vi "addItem.vi"(0 "reference in":refnum<class "Items Controller.lvclass">, 5 "dataIN":string[](array[string]), 7 "storageIN":string[][](array[string]), 11 "error in (no error)":errorcluster) -> (4 "reference out":refnum<class "Items Controller.lvclass">, 6 "found?":bool, 10 "storageOUT":string[][](array[string]), 15 "error out":errorcluster)   [LabVIEW 2014, in "Items Controller.lvclass"]
uses:
  Items Controller.lvclass
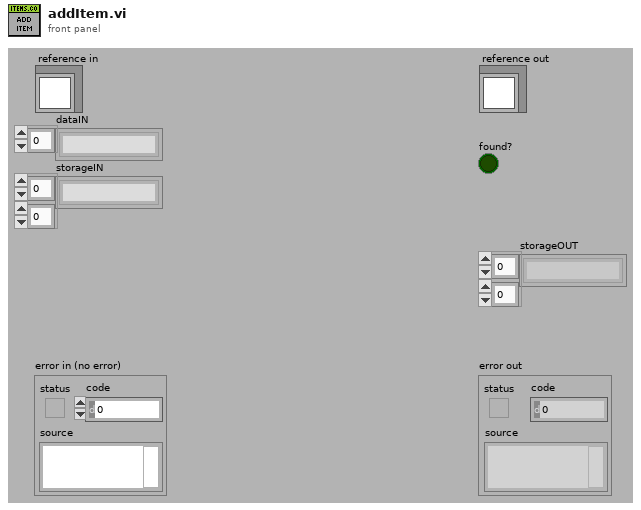
[diagram p1: front panel]
types:
  T1 = typedef "Items Controller.lvclass/ObjectAttributesRef.ctl" = refnum<data-value>
  T2 = typedef "Items Controller.lvclass/ObjectAttributes.ctl" = cluster{"MyAttribute":dbl, "data":string[][][], "file_controller_ref":refnum<class "File Controller.lvclass">, "checkIN_ref":refnum<class "checkIN.lvclass">, "checkOUT_ref":refnum<class "checkOUT.lvclass">, "item_ref":refnum<class "item.lvclass">}
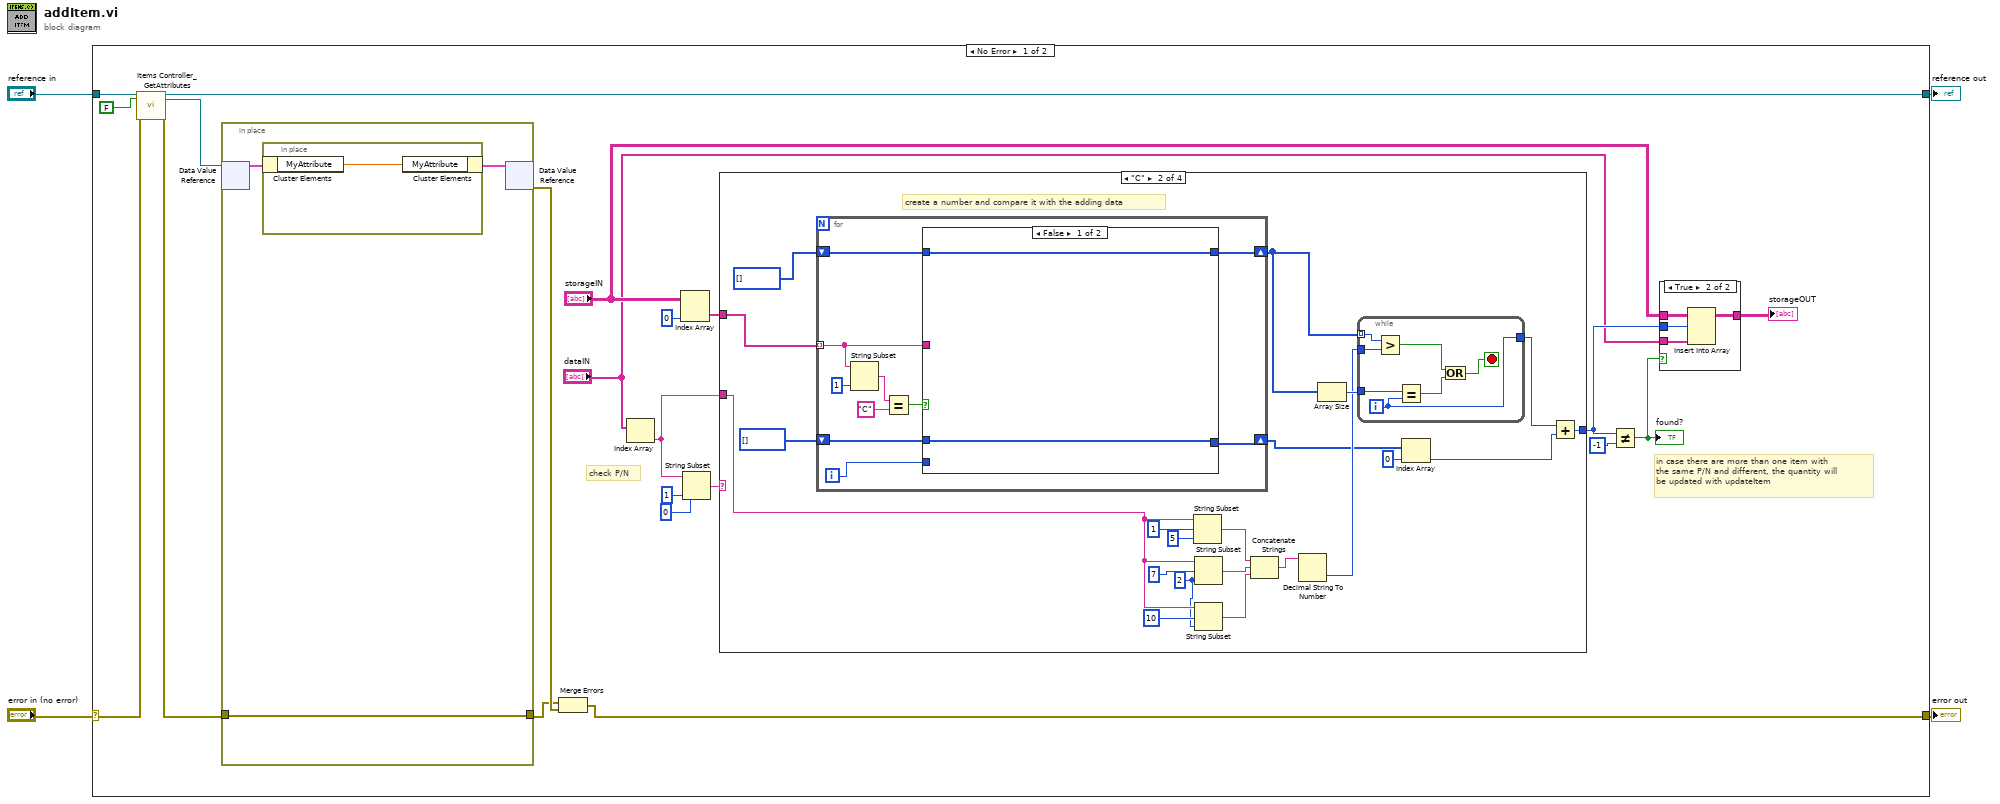
[diagram p0: block diagram]
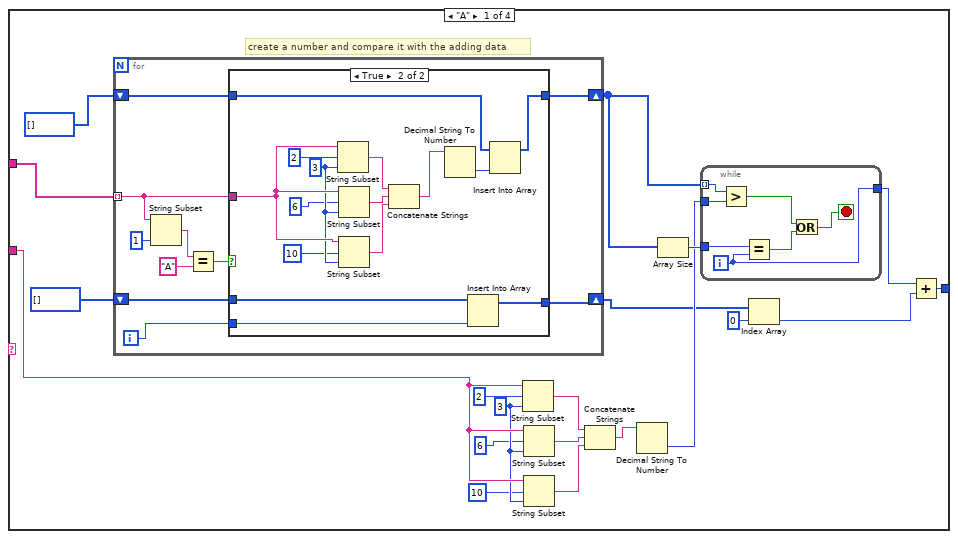
[diagram p3: hidden frame]
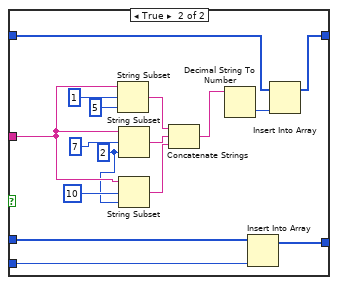
[diagram p5: hidden frame]
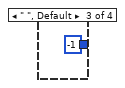
[diagram p6: hidden frame]
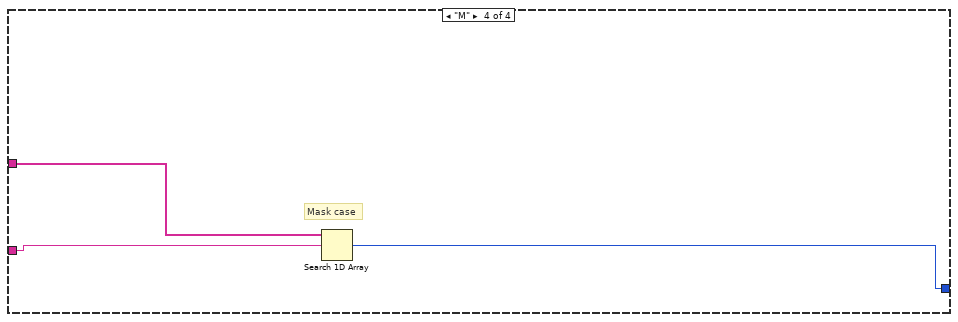
[diagram p7: hidden frame]
diagram:
  n1 = case shown="No Error" "error in (no error)" {
    selector: "error in (no error)" -> [w21 w150]
    tunnel: [w17 w150] -> w3
    tunnel: [w19 w149] -> w1
    tunnel: "reference in" -> [w23 w149]
    frame No Error {
      # "in case there are more than one item with\nthe same P/N and different, the quantity will\nbe updated with updateItem"
      # "check P/N"
      n2 = call "Items Controller_GetAttributes.vi"("reference in"=w23, "return data? (T)"=FALSE, "error in (no error)"=w21) -> ("reference out"=w19:refnum<class "Items Controller.lvclass">, "attributes ref"=w18:T1, "error out"=w20:errorcluster)  [unwired: 13 in, 1 out]
      n3 = in-place {
        in-place-border: w20 -> [w145]
        in-place-border: [w145] -> w24
        n4 = in-place-dvr #1(w18) -> (w146:T2)  [unwired: 1 out]
        n5 = in-place {
          n6 = in-place-cluster #2(w146) -> ("MyAttribute"=w148:dbl)
          n7 = in-place-cluster #2("MyAttribute"=w148) -> (w147:T2)
        }
        n8 = in-place-dvr #1(w147) -> (w25:errorcluster)  [unwired: 1 out]
      }
      n9 = Merge Errors(w24, w25) -> (w17:errorcluster)
      n10 = Index Array(array="dataIN") -> (element=w13:string)  [unwired: 1 in]
      n11 = Index Array(array="storageIN", index (col)=0 ("disabled index (col)")) -> (element=w12:string[])  [unwired: 1 in]
      n12 = String Subset(string=w13, offset (0)=0, length (rest)=1 ("length (rest)")) -> (substring=w14:string)
      n13 = case shown="\"C\"" w14 {
        tunnel: w13 -> [w50 w105 _ w143]
        tunnel: w12 -> [w49 w104 _ w144]
        tunnel: [w31 w86 -1 w142] -> w7
        frame "A" {
          w47 = 3 ("length (rest)")
          # "create a number and compare it with the adding data"
          n14 = for {
            tunnel: w49 -> [w64] mode=indexing
            shift-right: [w61] -> w38
            shift-left: i32[] [] -> [w62]
            shift-right: [w59] -> w35
            shift-left: i32[] [] -> [w60]
            i -> [w58]
            n15 = String Subset(string=w64, length (rest)=1 ("length (rest)")) -> (substring=w66:string)  [unwired: 1 in]
            n16 = Equal?(x=w66, y="A") -> (x = y?=w63:bool)
            n17 = case shown="True" w63 {
              tunnel: w64 -> [_ w84]
              tunnel: w62 -> [w69 w79]
              tunnel: [w69 w77] -> w61
              tunnel: w60 -> [w68 w74]
              tunnel: [w68 w76] -> w59
              tunnel: w58 -> [_ w75]
              frame False {
              }
              frame True {
                w82 = 3 ("length (rest)")
                n18 = String Subset(string=w84, offset (0)=2, length (rest)=w82) -> (substring=w72:string)
                n19 = String Subset(string=w84, offset (0)=6, length (rest)=w82) -> (substring=w73:string)
                n20 = String Subset(string=w84, offset (0)=10, length (rest)=w82) -> (substring=w71:string)
                n21 = Concatenate Strings(w72, w73, w71) -> (w70:string)
                n22 = Decimal String To Number(string=w70) -> (number=w78:i32)  [unwired: 2 in, 1 out]
                n23 = Insert Into Array(array=w74, new element=w75) -> (w76:i32[])  [unwired: 1 in]
                n24 = Insert Into Array(array=w79, new element=w78) -> (w77:i32[])  [unwired: 1 in]
              }
            }
          }
          n25 = String Subset(string=w50, offset (0)=2, length (rest)=w47) -> (substring=w42:string)
          n26 = String Subset(string=w50, offset (0)=6, length (rest)=w47) -> (substring=w41:string)
          n27 = String Subset(string=w50, offset (0)=10, length (rest)=w47) -> (substring=w40:string)
          n28 = Concatenate Strings(w42, w41, w40) -> (w39:string)
          n29 = Decimal String To Number(string=w39) -> (number=w36:i32)  [unwired: 2 in, 1 out]
          n30 = Array Size(array=w38) -> (size(s)=w37:i32)
          n31 = while {
            tunnel: w38 -> [w56] mode=indexing
            tunnel: w36 -> [w57]
            tunnel: [w55] -> w33
            tunnel: w37 -> [w54]
            i -> [w55]
            stop <- w52 stop-if-true
            n32 = Greater?(x=w56, y=w57) -> (0:w51:bool)
            n33 = Equal?(x=w54, y=w55) -> (x = y?=w53:bool)
            n34 = Or(x=w51, y=w53) -> (x .or. y?=w52:bool)
          }
          n35 = Index Array(array=w35, index=0) -> (element=w32:i32)
          n36 = Add(x=w33, y=w32) -> (x+y=w31:i32)
        }
        frame "C" {
          w85 = 2 ("length (rest)")
          # "create a number and compare it with the adding data"
          n37 = for {
            tunnel: w104 -> [w119] mode=indexing
            shift-right: [w116] -> w93
            shift-left: i32[] [] -> [w117]
            shift-right: [w114] -> w90
            shift-left: i32[] [] -> [w115]
            i -> [w113]
            n38 = String Subset(string=w119, length (rest)=1 ("length (rest)")) -> (substring=w121:string)  [unwired: 1 in]
            n39 = Equal?(x=w121, y="C") -> (x = y?=w118:bool)
            n40 = case shown="False" w118 {
              tunnel: w119 -> [_ w140]
              tunnel: w117 -> [w124 w135]
              tunnel: [w124 w133] -> w116
              tunnel: w115 -> [w123 w130]
              tunnel: [w123 w132] -> w114
              tunnel: w113 -> [_ w131]
              frame False {
              }
              frame True {
                w125 = 2 ("length (rest)")
                n41 = String Subset(string=w140, offset (0)=1, length (rest)=5 ("length (rest)")) -> (substring=w128:string)
                n42 = String Subset(string=w140, offset (0)=7, length (rest)=w125) -> (substring=w129:string)
                n43 = String Subset(string=w140, offset (0)=10, length (rest)=w125) -> (substring=w127:string)
                n44 = Concatenate Strings(w128, w129, w127) -> (w126:string)
                n45 = Decimal String To Number(string=w126) -> (number=w134:i32)  [unwired: 2 in, 1 out]
                n46 = Insert Into Array(array=w130, new element=w131) -> (w132:i32[])  [unwired: 1 in]
                n47 = Insert Into Array(array=w135, new element=w134) -> (w133:i32[])  [unwired: 1 in]
              }
            }
          }
          n48 = String Subset(string=w105, offset (0)=1, length (rest)=5 ("length (rest)")) -> (substring=w97:string)
          n49 = String Subset(string=w105, offset (0)=7, length (rest)=w85) -> (substring=w96:string)
          n50 = String Subset(string=w105, offset (0)=10, length (rest)=w85) -> (substring=w95:string)
          n51 = Concatenate Strings(w97, w96, w95) -> (w94:string)
          n52 = Decimal String To Number(string=w94) -> (number=w91:i32)  [unwired: 2 in, 1 out]
          n53 = Array Size(array=w93) -> (size(s)=w92:i32)
          n54 = while {
            tunnel: w93 -> [w111] mode=indexing
            tunnel: w91 -> [w112]
            tunnel: [w110] -> w88
            tunnel: w92 -> [w109]
            i -> [w110]
            stop <- w107 stop-if-true
            n55 = Greater?(x=w111, y=w112) -> (0:w106:bool)
            n56 = Equal?(x=w109, y=w110) -> (x = y?=w108:bool)
            n57 = Or(x=w106, y=w108) -> (x .or. y?=w107:bool)
          }
          n58 = Index Array(array=w90, index=0) -> (element=w87:i32)
          n59 = Add(x=w88, y=w87) -> (x+y=w86:i32)
        }
        frame " ", Default {
        }
        frame "M" {
          # "Mask case"
          n60 = Search 1D Array(1D array=w144, element=w143) -> (index of element=w142:i32)  [unwired: 1 in]
        }
      }
      n61 = Not Equal?(x=w7, y=-1) -> (x != y?=w6:bool)
      "found?" <- w6
      n62 = case shown="True" w6 {
        tunnel: "storageIN" -> [w26 w30]
        tunnel: [w26 w29] -> w8
        tunnel: "dataIN" -> [_ w28]
        tunnel: w7 -> [_ w27]
        frame False {
        }
        frame True {
          n63 = Insert Into Array(array=w30, index (row)=w27, new element=w28) -> (w29:string[][])  [unwired: 1 in]
        }
      }
      "storageOUT" <- w8
    }
    frame Error {
    }
  }
  "error out" <- w3
  "reference out" <- w1
